vi "Export.vi"(6 "Overwrite (F)":bool, 8 "error in (no error)":errorcluster, 9 "Experts":string, 10 "Destination File":path, 11 "Session in":refnum<k21>="localhost") -> (0 "error out":errorcluster, 3 "Session out":refnum<k21>)   [LabVIEW 2017, in "nisyscfg.lvlib"]
doc: "<B>NOTE:</B> This VI is a replacement for the deprecated MAX Copy Configuration.\n\nUse this VI to export configuration data from MAX into a file. Not all products are supported; consult your product documentation."
uses:
  <vilib>/nisyscfg/nisyscfg.lvlib
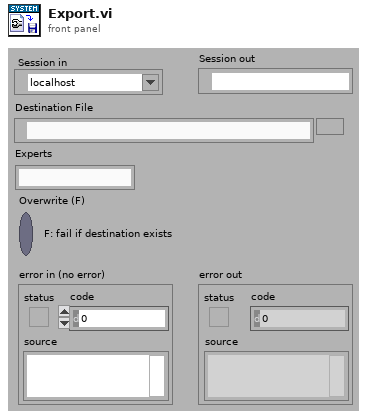
[diagram p1: front panel]
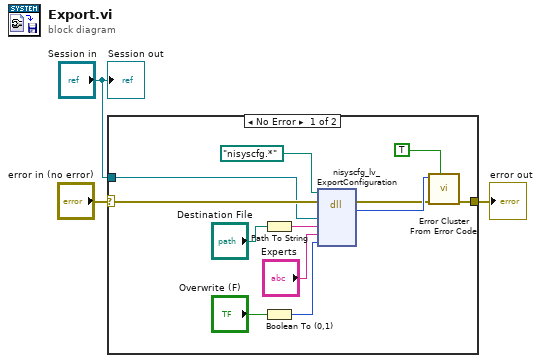
[diagram p0: block diagram]
diagram:
  n1 = case shown="No Error" "error in (no error)" {
    selector: "error in (no error)" -> [w7 w16]
    tunnel: [w14 w16] -> w3
    tunnel: "Session in" -> [w6 _]
    frame No Error {
      n2 = Path To String(path="Destination File") -> (string=w11:string)
      n3 = Boolean To (0,1)(Boolean="Overwrite (F)") -> (0, 1=w8:i16)
      n4 = dll-call lib="nisyscfg.*" fn="nisyscfg_lv_ExportConfiguration" label="ExportConfiguration"(path in=path "nisyscfg.*", error in=w7, "sessionHandle"=w6, "destinationFilename"=w11, "expertNames"="Experts", "overwriteIfExists"=w8) -> (error out=w12:errorcluster, "return type"=w13:i32)  [unwired: 5 in, 1 out]
      n5 = call <vilib>:"Error Cluster From Error Code.vi"("show call chain? (False)"=TRUE, "error in (no error)"=w12, "error code (0)"=w13) -> ("error out"=w14:errorcluster)  [unwired: 6 out]
    }
    frame Error {
    }
  }
  "error out" <- w3
  "Session out" <- "Session in"
